vi "Nonlinear Spring Constant fit.vi"() -> ()   [LabVIEW 2023]
doc: "Demonstrates fitting a parameterized simulation (ODE) using the Constrained Nonlinear Optimization VI. The system being simulated is a damped spring-mass system with a nonlinear (second order) spring. This example uses the optimization interface to implement a live update of a graph and control during the fitting process."
uses:
  <vilib>/gmath/NumericalOptimization/cno_bounds.ctl
  <vilib>/gmath/NI_Gmath.lvlib
panel:
  in  "Fit data?":bool
  in  "Stop":bool
  in  "spring constant":dbl(slide)=2.0 min=0.1 max=10.0 step=0.1 scale=0.1..10.0
  out "number of function calls":dbl
  in  "Initial Conditions":dbl[](array[numeric])=[1.0, 0.0]
  in  "xp Noise sigma":dbl(slide)=0.05 scale=0.0..0.1
  in  "spring constant (fit)":dbl(slide)=0.4 min=0.1 step=0.1 scale=0.1..4.0
  out "spring simulation":cluster{"times":dbl[], "outputs":dbl[]}[](graph)
  # "Overview: Demonstrates fitting a parameterized simulation (ODE) using the Constrained Nonlinear Optimization VI.  \nRequirements: LabVIEW Full Development System\nInstructions: \n1. Run the VI.\n2. Change the spring constant slider to have a value greater than 4.\n3. Click Fit Data, and notice that the identified spring constant has been limited. The spring constant has fitting bounds that are taken from range of the spring constant (fit) slider scale.\n4. Change the spring constant (fit) slider scale to have an upper limit of 10.\n5. Click Fit Data again and observe that the fit now has greater bounds.\n6. Click Stop to stop the VI."
  # "xp (position)"
  # "xv (velocity)"
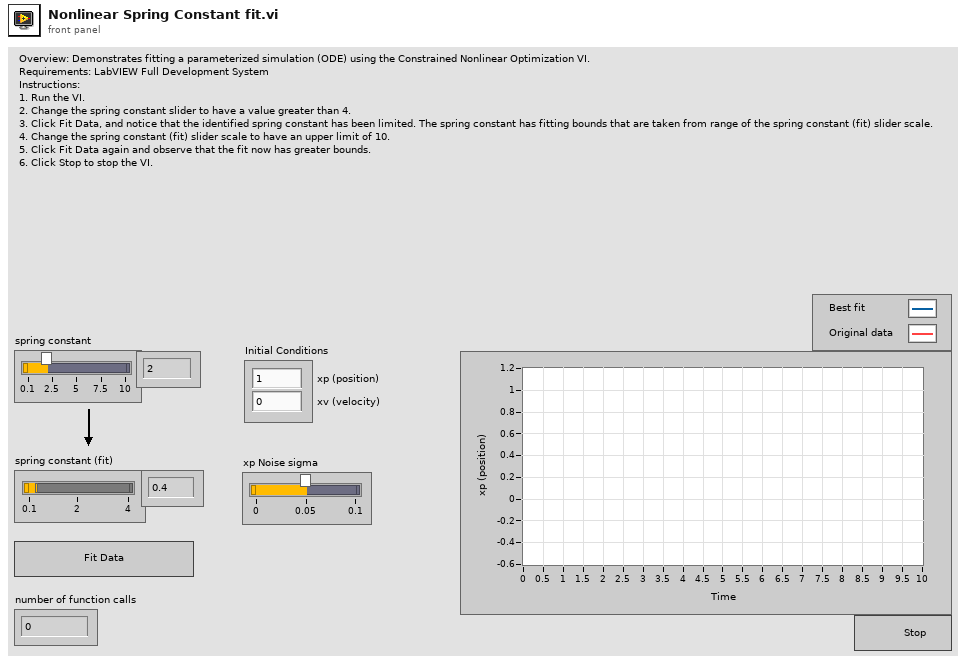
[diagram p1: front panel]
types:
  T1 = typedef "NI_Gmath.lvlib/cno_bounds.ctl" = cluster{"X minimum":dbl[], "X maximum":dbl[], "inequality constraint minimum":dbl[], "inequality constraint maximum":dbl[]}
  T2 = cluster{"function tolerance":dbl, "parameter tolerance":dbl, "max iterations":i32, "max function calls":i32, "gradient tolerance":dbl, "max time (sec)":dbl}
  T3 = cluster{"Initial Time":dbl, "Final Time":dbl, "Time Step":dbl, "Absolute Tolerance":dbl, "Relative Tolerance":dbl, "Solver Method":enum16{"Runge-Kutta 1 (Euler)", "Runge-Kutta 2", "Runge-Kutta 3", "Runge-Kutta 4", "Runge-Kutta 23 (variable)", "Runge-Kutta 45 (variable)", "BDF (variable)", "Adams-Moulton (variable)", "Rosenbrock (variable)", "Discrete States Only"}, "Discrete Time Step":dbl, "Minimum Time Step":dbl, "Maximum Time Step":dbl, "Initial Time Step":dbl}
  T4 = cluster{"outputs":dbl[][], "times":dbl[], "Initial Conditions":dbl[], "ODE Solver Parameters":cluster{"Initial Time":dbl, "Final Time":dbl, "Time Step":dbl, "Absolute Tolerance":dbl, "Relative Tolerance":dbl, "Solver Method":enum16{"Runge-Kutta 1 (Euler)", "Runge-Kutta 2", "Runge-Kutta 3", "Runge-Kutta 4", "Runge-Kutta 23 (variable)", "Runge-Kutta 45 (variable)", "BDF (variable)", "Adams-Moulton (variable)", "Rosenbrock (variable)", "Discrete States Only"}, "Discrete Time Step":dbl, "Minimum Time Step":dbl, "Maximum Time Step":dbl, "Initial Time Step":dbl}, "spring simulation":refnum<vi>, "spring constant (fit)":refnum<vi>}
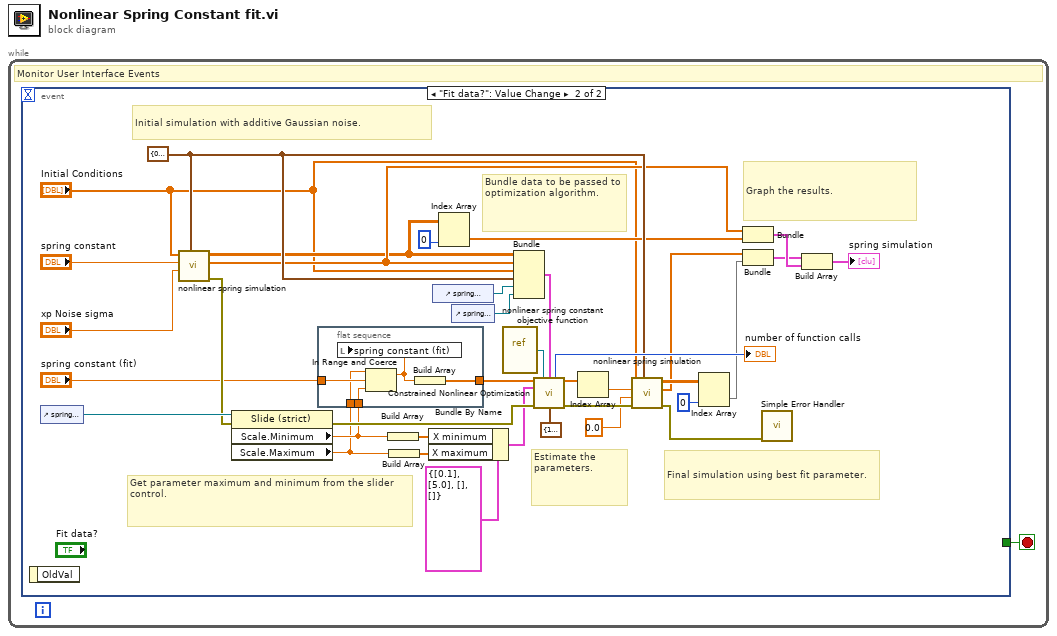
[diagram p0: block diagram]
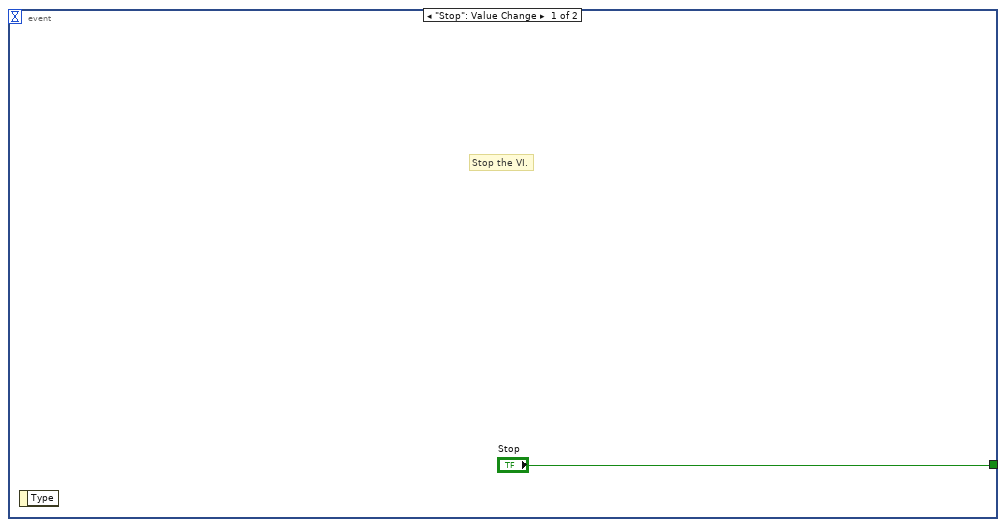
[diagram p2: hidden frame]
diagram:
  n1 = while {
    stop <- w1 stop-if-true
    # "Monitor User Interface Events"
    n2 = event shown="[1] \"Fit data?\": Value Change" {
      selector: _ -> [_ _]
      dyn-events: _ -> [_ _]
      timeout: _ -> [_ _]
      tunnel: ["Stop" _] -> w1
      event "Stop": Value Change {
        # "Stop the VI."
        n3 = event-data() -> ()  [unwired: 1 in, 1 out]
      }
      event "Fit data?": Value Change {
        w32 = T3 {"Initial Time"=0.0, "Final Time"=10.0, "Time Step"=0.1, "Absolute Tolerance"=0.001, "Relative Tolerance"=1e-07, "Solver Method"=enum."Runge-Kutta 45 (variable)", "Discrete Time Step"=0.1, "Minimum Time Step"=0.01, "Maximum Time Step"=0.1, "Initial Time Step"=0.01} ("ODE Solver Parameters")
        # "Graph the results."
        # "Bundle data to be passed to optimization algorithm."
        # "Initial simulation with additive Gaussian noise."
        # "Final simulation using best fit parameter."
        # "Get parameter maximum and minimum from the slider control."
        # "Estimate the parameters."
        n4 = event-data() -> ()  [unwired: 1 in, 1 out]
        n5 = control-ref of="spring constant (fit)"() -> (w20:refnum<vi>)
        n6 = call "nonlinear spring simulation.vi"("Solver Params"=w32, "xp Noise STD"="xp Noise sigma", "Spring Constant"="spring constant", "Initial Conditions"="Initial Conditions") -> ("Error Out"=w10:errorcluster, "times"=w18:dbl[], "outputs"=w16:dbl[][])  [unwired: 5 in]
        n7 = property class="Slide (strict)"(reference=w20, error in=w10) -> (error out=w9:errorcluster, "Scale.Minimum"=w4:dbl, "Scale.Maximum"=w3:dbl)  [unwired: 1 out]
        n8 = flat-sequence {
          tunnel: [w44] -> w24
          tunnel: "spring constant (fit)" -> [w43]
          tunnel: w4 -> [w42]
          tunnel: w3 -> [w41]
          frame #0 {
            n9 = In Range and Coerce(upper limit=w41, x=w43, lower limit=w42) -> (coerced(x)=w40:dbl)  [unwired: 1 out]
            n10 = local write "spring constant (fit)"(w40) -> ()
            n11 = Build Array(w40) -> (w44:dbl[])
          }
        }
        n12 = Build Array(w4) -> (w21:dbl[])
        n13 = Build Array(w3) -> (w22:dbl[])
        n14 = Bundle By Name(cluster=T1 {"X minimum"=[0.1], "X maximum"=[5.0], "inequality constraint minimum"=[], "inequality constraint maximum"=[]} ("bounds"), "X minimum"=w21, "X maximum"=w22) -> (w6:T1)
        n15 = control-ref of="spring simulation"() -> (w33:refnum<vi>)
        n16 = Index Array(array=w16, index (col)=0 ("disabled index (col)")) -> (element=w17:dbl[])  [unwired: 1 in]
        n17 = control-ref of="spring constant (fit)"() -> (w38:refnum<vi>)
        n18 = vi-ref "nonlinear spring constant objective function.vi"() -> (w14:refnum<vi>)
        n19 = Bundle("outputs"=w16, "times"=w18, "Initial Conditions"="Initial Conditions", "ODE Solver Parameters"=w32, "spring simulation"=w33, "spring constant (fit)"=w38) -> (w13:T4)  [unwired: 1 in]
        n20 = call <vilib>:"Constrained Nonlinear Optimization.vi"("start"=w24, "objective and constraint function"=w14, "function data"=w13, "bounds"=w6, "error in (no error)"=w9, "stopping criteria"=T2 {"function tolerance"=1e-06, "parameter tolerance"=1e-06, "max iterations"=100, "max function calls"=1000, "gradient tolerance"=1e-06, "max time (sec)"=-1.0}) -> ("number of function calls"=→"number of function calls":i32, "minimum"=w25:dbl[], "error out"=w31:errorcluster)  [unwired: 5 in, 2 out]
        n21 = Index Array(array=w25) -> (element=w36:dbl)  [unwired: 1 in]
        n22 = call "nonlinear spring simulation.vi"("Solver Params"=w32, "Error In"=w31, "xp Noise STD"=0.0, "Spring Constant"=w36, "Initial Conditions"="Initial Conditions") -> ("Error Out"=w11:errorcluster, "times"=w27:dbl[], "outputs"=w29:dbl[][])  [unwired: 4 in]
        n23 = Index Array(array=w29, index (col)=0 ("disabled index (col)")) -> (element=w30:dbl[])  [unwired: 1 in]
        n24 = Bundle("times"=w18, "outputs"=w17) -> (w35:cluster{"times":dbl[], "outputs":dbl[]})  [unwired: 1 in]
        n25 = Bundle("times"=w27, "outputs"=w30) -> (w34:cluster{"times":dbl[], "outputs":dbl[]})  [unwired: 1 in]
        n26 = call <vilib>:"Simple Error Handler.vi"("error in (no error)"=w11) -> ()  [unwired: 4 in, 5 out]
        n27 = Build Array(w34, w35) -> (→"spring simulation":cluster{"times":dbl[], "outputs":dbl[]}[])
      }
    }
  }
